vi "Config Data Write To File.vi"(8 "error in (no error)":errorcluster caption="Fehler (Eingang, kein Fehler)", 11 "config data reference":T1 caption="Konfigurationsdaten-Referenz") -> (0 "error out":errorcluster caption="Fehler (Ausgang)", 3 "config data reference out":T1 caption="Konfigurationsdaten-Referenz (Ausgang)")   [LabVIEW 2009]
doc: "Schreibt die Daten aus dem Konfigurationsdaten-Objekt, in die Konfigurationsdatei, die in der Objekteigenschaft \"Dateipfad\" angegeben ist. Wenn die Eigenschaft \"Pfad\" keinen Pfad enthält, macht dieses VI nichts. Wenn der Schlüssel nicht existiert, wird vom VI ein Fehler ausgegeben."
uses:
  <vilib>/Utility/config.llb/Config Data RefNum.ctl
  Config Data Registry Functions.ctl
  <vilib>/Utility/config.llb/NI_LVConfig.lvlib
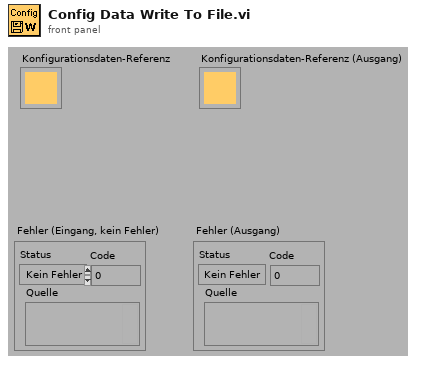
[diagram p1: front panel]
types:
  T1 = typedef "NI_LVConfig.lvlib/Config Data RefNum.ctl" = refnum<k1>
  T2 = typedef "Config Data Registry Functions.ctl" = enum16{"reset", "register", "get data", "get section", "set data", "unregister", "test", "get objects"}
  T3 = typedef "Config Data.ctl" = cluster{"file path":path, "data":T4[], "section names":string[]}
  T4 = typedef "Config Data Section.ctl" = cluster{"keys":string[], "values":string[]}
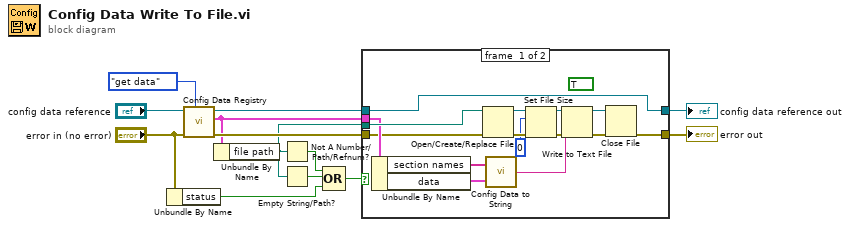
[diagram p0: block diagram]
diagram:
  n1 = Unbundle By Name("error in (no error)") -> ("status"=w5:bool)
  n2 = call "Config Data Registry.vi"("function (get data)"=Config_Data_Registry_Functions."get data", "error in (no error)"="error in (no error)", "config data"="config data reference") -> ("error out"=w8:errorcluster, 2:"config data out"=w2:T3, 3:"config data out"=w9:T1)  [unwired: 2 in, 4 out]
  n3 = Unbundle By Name(w2) -> ("file path"=w3:path)
  n4 = Not A Number/Path/Refnum?(number/path/refnum=w3) -> (NaN/Path/Refnum?=w6:bool)
  n5 = Empty String/Path?(string/path=w3) -> (empty?=w7:bool)
  n6 = Compound Arithmetic op=OR(w6, w7, w5) -> (w4:bool)
  n7 = case shown="False" w4 {
    tunnel: w9 -> [w24 w29]
    tunnel: w8 -> [w21 w30]
    tunnel: [w24 w29] -> w13
    tunnel: [w26 w30] -> w12
    tunnel: w3 -> [w23 _]
    tunnel: w2 -> [w22 _]
    frame #0 {
      (unwired) TRUE ("convert eol (F)")
      n8 = Unbundle By Name(w22) -> ("section names"=w15:string[], "data"=w25:T4[])
      n9 = Open/Create/Replace File(file path (use dialog)=w23, error in=w21) -> (refnum out=w17:refnum<file>, error out=w20:errorcluster)  [unwired: 4 in, 1 out]
      n10 = call "Config Data to String.vi"("data"=w25, "section names"=w15) -> ("string"=w14:string)
      n11 = Set File Size(4:w20, 6:0 ("pos offset (0)"), 7:w17) -> (0:w19:errorcluster, 3:w18:refnum<file>)
      n12 = Write to Text File(file (use dialog)=w18, text=w14, error in=w19) -> (refnum out=w28:refnum<file>, error out=w27:errorcluster)  [unwired: 1 in, 1 out]
      n13 = Close File(refnum=w28, error in=w27) -> (error out=w26:errorcluster)  [unwired: 1 out]
    }
    frame #1 {
    }
  }
  "error out" <- w12
  "config data reference out" <- w13
